vi "ITC4005_Init_config_current_mode.vi"(0 "VISA ITC4005":refnum<visa-resource-name>="USB0::0x1313::0x804A::M00324116::INSTR" caption="resource name", 2 "T Protection Mode\n (Disabled (No function))":i16(ring)=1 caption="Mode (Disabled (No function))" items=["Disabled (No function)", "Output Enable", "Output Protection"], 5 "General LD Configuration":T3={"Laser Diode Operating Mode (Constant Current)"=0, "Laser Diode Current Limit (0.0)"=1.0} {"Laser Diode Operating Mode (Constant Current)" items=["Constant Current", "Constant Power"]}, 7 "Laser diode output":T2={"Delay (1.0)"=1.0, "LD Voltage Limit (6.0)"=6.0}, 9 "TEC Settings":T1={"TEC Operating Mode (Constant Temperature)"=1, "TEC Temperature Setpoint (20.0)"=20.0} {"TEC Operating Mode (Constant Temperature)" items=["Constant Temperature"=1, "Current Source"=0]}, 11 "error in":errorcluster) -> (4 "ITC4005 handle out":refnum<visa-resource-name>="USB0::0x1313::0x804A::M00324116::INSTR" caption="instrument handle out", 15 "error out":errorcluster)   [LabVIEW 2019]
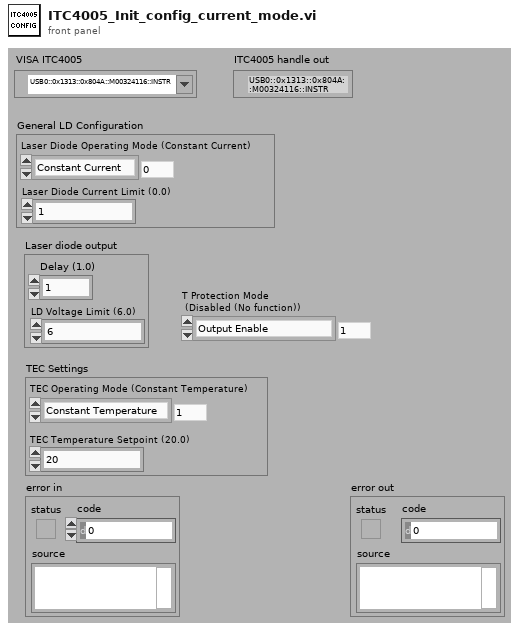
[diagram p1: front panel]
types:
  T1 = cluster{"TEC Operating Mode (Constant Temperature)":i16, "TEC Temperature Setpoint (20.0)":dbl}
  T2 = cluster{"Delay (1.0)":dbl, "LD Voltage Limit (6.0)":dbl}
  T3 = cluster{"Laser Diode Operating Mode (Constant Current)":i16, "Laser Diode Current Limit (0.0)":dbl}
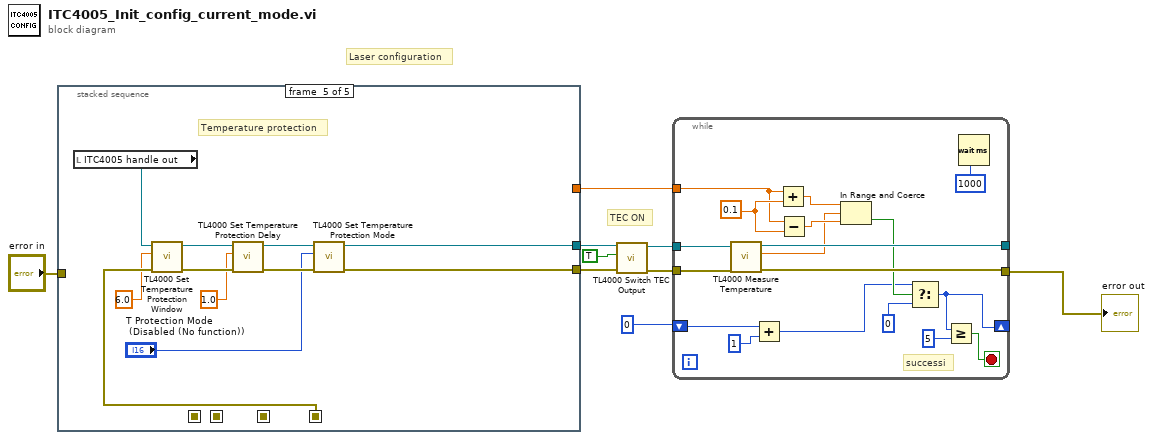
[diagram p0: block diagram]
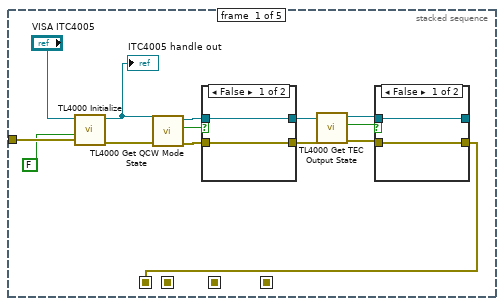
[diagram p2: hidden frame]
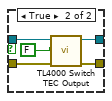
[diagram p3: hidden frame]
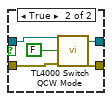
[diagram p4: hidden frame]
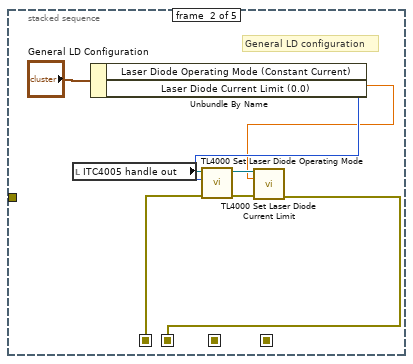
[diagram p5: hidden frame]
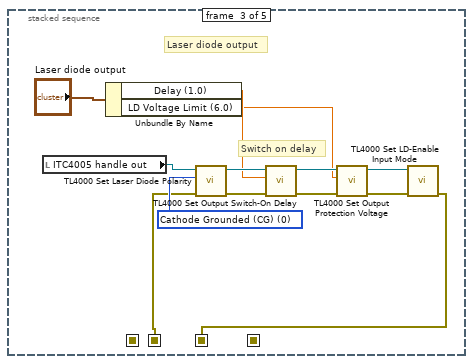
[diagram p6: hidden frame]
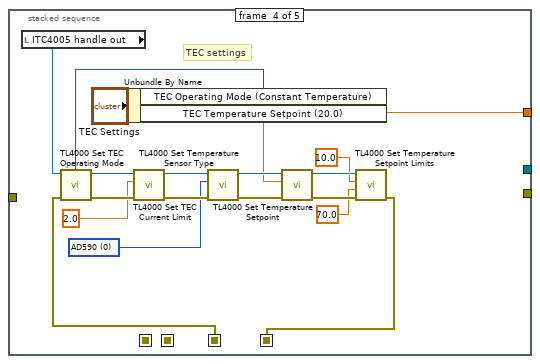
[diagram p7: hidden frame]
diagram:
  # "Laser configuration"
  # "TEC ON"
  n1 = stacked-sequence {
    seq-local: [w10 _ _ _ _] -> [_ w44 _ _ _]
    seq-local: [_ w38 _ _ _] -> [_ _ w46 _ _]
    seq-local: [_ _ w50 _ _] -> [_ _ _ w59 _]
    seq-local: [_ _ _ w70 _] -> [_ _ _ _ w87]
    tunnel: "error in" -> [w23 _ _ _ _]
    tunnel: [_ _ _ _ w78] -> w4
    tunnel: [_ _ _ _ w77] -> w5
    tunnel: [_ _ _ w60 _] -> w3
    frame #0 {
      n2 = call "TL4000 Initialize.vi"("error in (no error)"=w23, "Reset Device (Reset Device)"=FALSE, "resource name"="VISA ITC4005") -> ("error out"=w19:errorcluster, "instrument handle out"=w20:refnum<visa-resource-name>)  [unwired: 7 in]
      "ITC4005 handle out" <- w20
      n3 = call "TL4000 Get QCW Mode State.vi"("error in (no error)"=w19, "instrument handle"=w20) -> ("error out"=w16:errorcluster, "QCW Mode State"=w18:bool, "instrument handle out"=w17:refnum<visa-resource-name>)  [unwired: 7 in]
      n4 = case shown="False" w18 {
        tunnel: w17 -> [w32 w36]
        tunnel: w16 -> [w31 w35]
        tunnel: [w32 w34] -> w14
        tunnel: [w31 w33] -> w15
        frame False {
        }
        frame True {
          n5 = call "TL4000 Switch QCW Mode.vi"("error in (no error)"=w35, "QCW Mode (Off)"=FALSE, "instrument handle"=w36) -> ("error out"=w33:errorcluster, "instrument handle out"=w34:refnum<visa-resource-name>)  [unwired: 7 in]
        }
      }
      n6 = call "TL4000 Get TEC Output State.vi"("error in (no error)"=w15, "instrument handle"=w14) -> ("error out"=w11:errorcluster, "TEC Output"=w13:bool, "instrument handle out"=w12:refnum<visa-resource-name>)  [unwired: 7 in]
      n7 = case shown="False" w13 {
        tunnel: w12 -> [w25 w29]
        tunnel: w11 -> [w24 w27]
        tunnel: [w25 w26] -> _
        tunnel: [w24 w30] -> w10
        frame False {
        }
        frame True {
          n8 = call "TL4000 Switch TEC Output.vi"("error in (no error)"=w27, "TEC Output (Off)"=FALSE ("QCW Mode (Off)"), "instrument handle"=w29) -> ("error out"=w30:errorcluster, "instrument handle out"=w26:refnum<visa-resource-name>)  [unwired: 7 in]
        }
      }
    }
    frame #1 {
      # "General LD configuration"
      n9 = local read "ITC4005 handle out"() -> (w45:refnum<visa-resource-name>)
      n10 = Unbundle By Name("General LD Configuration") -> ("Laser Diode Operating Mode (Constant Current)"=w40:i16, "Laser Diode Current Limit (0.0)"=w39:dbl)
      n11 = call "TL4000 Set Laser Diode Operating Mode.vi"("error in (no error)"=w44, "Laser Diode Operating Mode (Constant Current)"=w40, "instrument handle"=w45) -> ("error out"=w43:errorcluster, "instrument handle out"=w42:refnum<visa-resource-name>)  [unwired: 7 in]
      n12 = call "TL4000 Set Laser Diode Current Limit.vi"("error in (no error)"=w43, "Laser Diode Current Limit (0.0)"=w39, "instrument handle"=w42) -> ("error out"=w38:errorcluster)  [unwired: 7 in, 1 out]
    }
    frame #2 {
      w51 = i16 0 items=["Cathode Grounded (CG)", "Anode Grounded (AG)"] ("Polarity (Cathode Grounded (CG))")
      # "Switch on delay"
      # "Laser diode output"
      n13 = local read "ITC4005 handle out"() -> (w58:refnum<visa-resource-name>)
      n14 = Unbundle By Name("Laser diode output") -> ("Delay (1.0)"=w48:dbl, "LD Voltage Limit (6.0)"=w47:dbl)
      n15 = call "TL4000 Set Laser Diode Polarity.vi"("error in (no error)"=w46, "Polarity (Cathode Grounded (CG))"=w51, "instrument handle"=w58) -> ("error out"=w57:errorcluster, "instrument handle out"=w56:refnum<visa-resource-name>)  [unwired: 7 in]
      n16 = call "TL4000 Set Output Switch-On Delay.vi"("error in (no error)"=w57, "Delay (1.0)"=w48, "instrument handle"=w56) -> ("error out"=w55:errorcluster, "instrument handle out"=w54:refnum<visa-resource-name>)  [unwired: 7 in]
      n17 = call "TL4000 Set Output Protection Voltage.vi"("error in (no error)"=w55, "Voltage (5.0)"=w47, "instrument handle"=w54) -> ("error out"=w53:errorcluster, "instrument handle out"=w52:refnum<visa-resource-name>)  [unwired: 7 in]
      n18 = call "TL4000 Set LD-Enable Input Mode.vi"("error in (no error)"=w53, "instrument handle"=w52) -> ("error out"=w50:errorcluster)  [unwired: 8 in, 1 out]
    }
    frame #3 {
      w65 = i16 0 items=["AD590", "Thermistor (low range)", "Thermistor (high range)", "PT100", "PT1000", "LM35", "LM335"] ("Sensor (AD590)")
      # "TEC settings"
      n19 = local read "ITC4005 handle out"() -> (w76:refnum<visa-resource-name>)
      n20 = Unbundle By Name("TEC Settings") -> ("TEC Operating Mode (Constant Temperature)"=w61:i16, "TEC Temperature Setpoint (20.0)"=w60:dbl)
      n21 = call "TL4000 Set TEC Operating Mode.vi"("error in (no error)"=w59, "TEC Operating Mode (Constant Temperature)"=w61, "instrument handle"=w76) -> ("error out"=w74:errorcluster, "instrument handle out"=w75:refnum<visa-resource-name>)  [unwired: 7 in]
      n22 = call "TL4000 Set TEC Current Limit.vi"("error in (no error)"=w74, "TEC Current Limit (1.0)"=2.0, "instrument handle"=w75) -> ("error out"=w73:errorcluster, "instrument handle out"=w69:refnum<visa-resource-name>)  [unwired: 7 in]
      n23 = call "TL4000 Set Temperature Sensor Type.vi"("error in (no error)"=w73, "Sensor (AD590)"=w65, "instrument handle"=w69) -> ("error out"=w72:errorcluster, "instrument handle out"=w68:refnum<visa-resource-name>)  [unwired: 7 in]
      n24 = call "TL4000 Set Temperature Setpoint.vi"("error in (no error)"=w72, "Temperature Setpoint (25.0)"=w60, "instrument handle"=w68) -> ("error out"=w71:errorcluster, "instrument handle out"=w67:refnum<visa-resource-name>)  [unwired: 7 in]
      n25 = call "TL4000 Set Temperature Setpoint Limits.vi"("error in (no error)"=w71, "Setpoint High Limit (50.0)"=70.0, "Setpoint Low Limit (0.0)"=10.0, "instrument handle"=w67) -> ("error out"=w70:errorcluster)  [unwired: 6 in, 1 out]
    }
    frame #4 {
      # "Temperature protection"
      n26 = local read "ITC4005 handle out"() -> (w85:refnum<visa-resource-name>)
      n27 = call "TL4000 Set Temperature Protection Window.vi"("error in (no error)"=w87, "Window (5.0)"=6.0, "instrument handle"=w85) -> ("error out"=w86:errorcluster, "instrument handle out"=w83:refnum<visa-resource-name>)  [unwired: 7 in]
      n28 = call "TL4000 Set Temperature Protection Delay.vi"("error in (no error)"=w86, "Delay (1.0)"=1.0, "instrument handle"=w83) -> ("error out"=w81:errorcluster, "instrument handle out"=w82:refnum<visa-resource-name>)  [unwired: 7 in]
      n29 = call "TL4000 Set Temperature Protection Mode.vi"("error in (no error)"=w81, "Mode (Disabled (No function))"="T Protection Mode\n (Disabled (No function))", "instrument handle"=w82) -> ("error out"=w78:errorcluster, "instrument handle out"=w77:refnum<visa-resource-name>)  [unwired: 7 in]
    }
  }
  n30 = call "TL4000 Switch TEC Output.vi"("error in (no error)"=w4, "TEC Output (Off)"=TRUE, "instrument handle"=w5) -> ("error out"=w7:errorcluster, "instrument handle out"=w8:refnum<visa-resource-name>)  [unwired: 7 in]
  n31 = while {
    tunnel: w7 -> [w104]
    tunnel: w8 -> [w105]
    tunnel: [w103] -> w1
    tunnel: [w102] -> _
    shift-right: [w93] -> _
    shift-left: 0 -> [w97]
    tunnel: w3 -> [w88]
    stop <- w94 stop-if-true
    w89 = 0.1 ("y")
    # "successi"
    n32 = call "TL4000 Measure Temperature.vi"("error in (no error)"=w104, "instrument handle"=w105) -> ("error out"=w103:errorcluster, "Temperature"=w99:dbl, "instrument handle out"=w102:refnum<visa-resource-name>)  [unwired: 7 in]
    n33 = Add(x=w97, y=1) -> (x+y=w95:i32)
    n34 = Add(x=w88, y=w89) -> (x+y=w100:dbl)
    n35 = Subtract(x=w88, y=w89) -> (x-y=w101:dbl)
    n36 = In Range and Coerce(upper limit=w100, x=w99, lower limit=w101) -> (In Range?=w98:bool)  [unwired: 1 out]
    n37 = Select(t=w95, s=w98, f=0) -> (s? t:f=w93:i32)
    n38 = Greater Or Equal?(x=w93, y=5) -> (x >= y?=w94:bool)
    n39 = Wait (ms)(milliseconds to wait=u32 1000) -> ()  [unwired: 1 out]
  }
  "error out" <- w1
